vi "Get Objects not in Range.vi"(8 "error in":errorcluster, 9 "Upper Bound":u16 format="%.0x", 10 "Lower Bound":u16 format="%.0x", 11 "Sorted Object Dictionary in":refnum<class "Sorted Object Dictionary.lvclass">) -> (0 "error out":errorcluster, 2 "Entries":refnum<class "OD Entry.lvclass">[](array[class]), 3 "Sorted Object Dictionary out":refnum<class "Sorted Object Dictionary.lvclass">)   [LabVIEW 2020, in "Electronic Datasheet.lvlib" / "Sorted Object Dictionary.lvclass"]
uses:
  Sorted Object Dictionary.lvclass
  Sorted Object Dictionary.lvclass/Sorted Object Dictionary.ctl
  Electronic Datasheet.lvlib
  OD Entry/OD Entry.lvclass
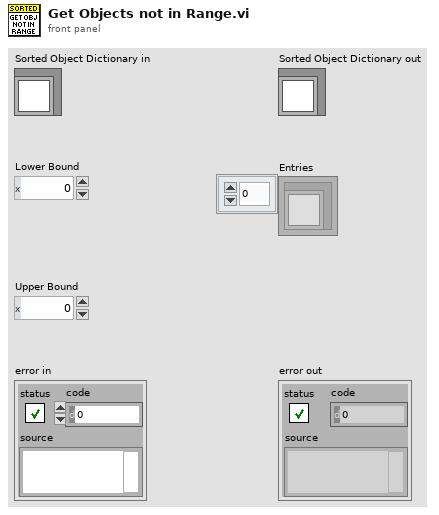
[diagram p1: front panel]
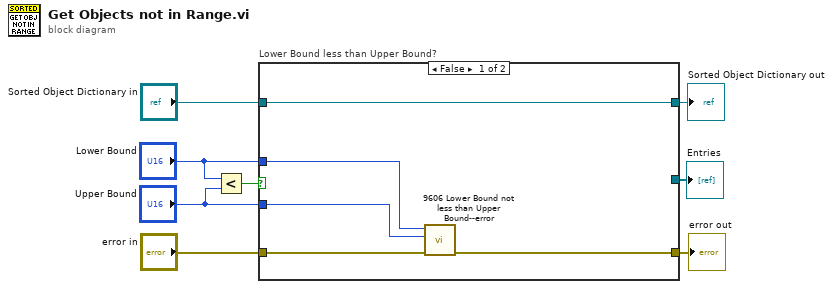
[diagram p0: block diagram]
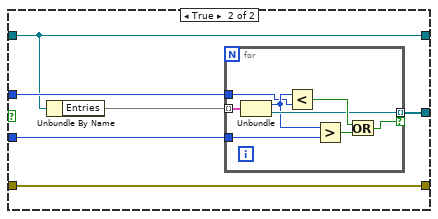
[diagram p2: hidden frame]
diagram:
  n1 = Less?(x="Lower Bound", y="Upper Bound") -> (x < y?=w3:bool)
  n2 = case "Lower Bound less than Upper Bound?" shown="False" w3 {
    tunnel: "Sorted Object Dictionary in" -> [w12 w14]
    tunnel: "Lower Bound" -> [w10 w19]
    tunnel: "Upper Bound" -> [w9 w17]
    tunnel: [_ w16] -> w7
    tunnel: "error in" -> [w11 w15]
    tunnel: [w13 w15] -> w2
    tunnel: [w12 w14] -> w1
    frame False {
      n3 = call "9606 Lower Bound not less than Upper Bound--error.vi"("error in"=w11, "Upper Bound"=w9, "Lower Bound"=w10) -> ("error out"=w13:errorcluster)  [unwired: 8 in]
    }
    frame True {
      n4 = Unbundle By Name(w14) -> ("Entries"=w18:map{u16, refnum<class "OD Entry.lvclass">})
      n5 = for {
        tunnel: w18 -> [w27] mode=indexing
        tunnel: w19 -> [w20]
        tunnel: w17 -> [w26]
        tunnel: [w23] -> w16 mode=indexing if=w22
        n6 = Unbundle(w27) -> ("Index"=w21:u16, "OD Entry"=w23:refnum<class "OD Entry.lvclass">)
        n7 = Less?(x=w21, y=w20) -> (x < y?=w24:bool)
        n8 = Greater?(x=w21, y=w26) -> (0:w25:bool)
        n9 = Or(x=w24, y=w25) -> (x .or. y?=w22:bool)
      }
    }
  }
  "error out" <- w2
  "Sorted Object Dictionary out" <- w1
  "Entries" <- w7
